vi "Drive_Auto_Module.vi"(5 "Y":dbl, 6 "Delay (s)":dbl, 7 "X":dbl, 11 "DevRef&Err":T7) -> (3 "DevRef&Err":T7)   [LabVIEW 2017]
uses:
  <vilib>/Rock Robotics/WPI/RobotDrive/WPI_RobotDriveDevRef.ctl
  <vilib>/Rock Robotics/WPI/MotorControl/WPI_MotorControlDeviceRef.ctl
  <vilib>/Rock Robotics/WPI/MotorControl/WPI_MotorControlType.ctl
  <vilib>/Rock Robotics/SystemInterfaces/DIO/FPGA_DIOPWMChannel.ctl
  <vilib>/Rock Robotics/WPI/PWM/WPI_PWMDeadband.ctl
  <vilib>/Rock Robotics/SystemInterfaces/DIO/FPGA_DIOChannel.ctl
  <vilib>/Rock Robotics/WPI/RobotDrive/WPI_RobotDriveMecanumDrive_Cartesian.vi
  <vilib>/Rock Robotics/Network Tables/NT Write Numeric Array.vi
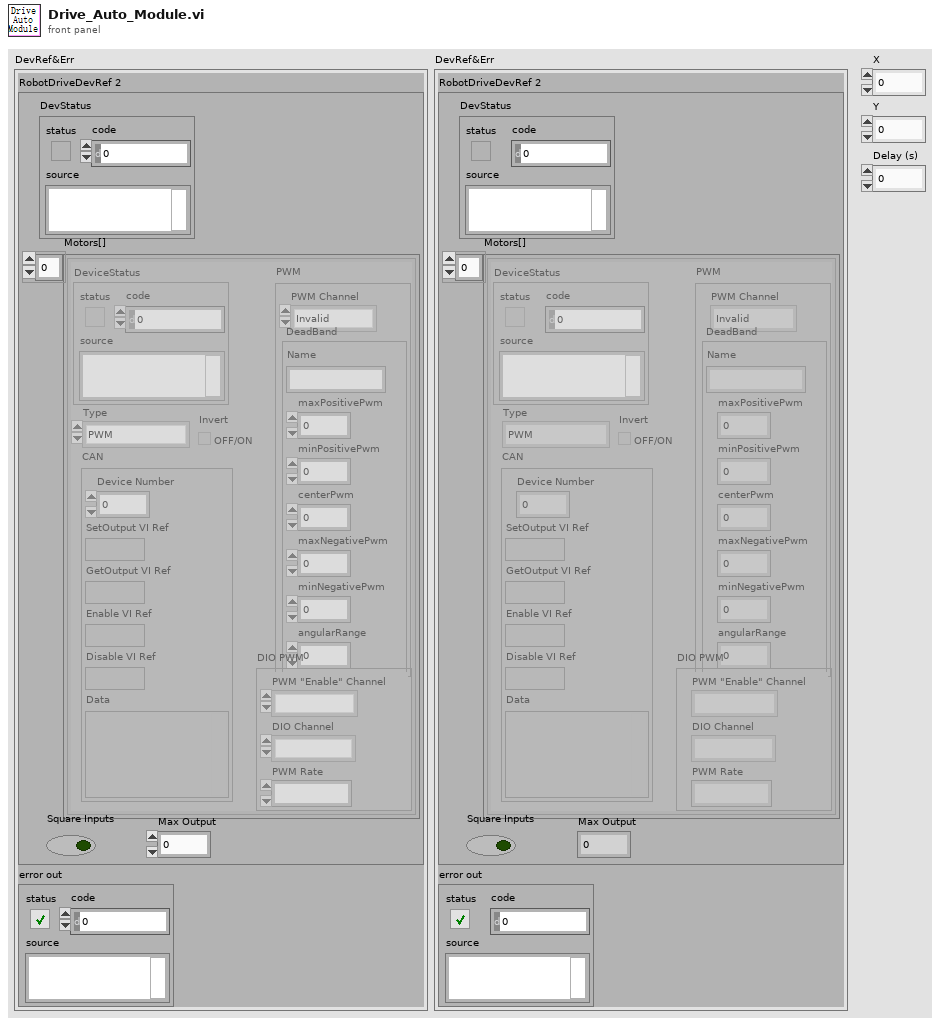
[diagram p1: front panel]
types:
  T1 = typedef "WPI_RobotDriveDevRef.ctl" = cluster{"DevStatus":errorcluster, "Motors[]":T2[], "Square Inputs":bool, "Max Output":dbl}
  T2 = typedef "WPI_MotorControlDeviceRef.ctl" = cluster{"DeviceStatus":errorcluster, "Type":T3, "PWM":cluster{"PWM Channel":T4, "DeadBand":T5}, "CAN":cluster{"Device Number":u8, "SetOutput VI Ref":variant, "GetOutput VI Ref":variant, "Enable VI Ref":variant, "Disable VI Ref":variant, "Data":variant}, "Invert":bool, "DIO PWM":cluster{"PWM \"Enable\" Channel":T4, "DIOChannel":T6, "PWM Rate":dbl}}
  T3 = typedef "WPI_MotorControlType.ctl" = enum16{"PWM", "CAN", "DIO PWM"}
  T4 = typedef "FPGA_DIOPWMChannel.ctl" = enum8{"PWM 0", "PWM 1", "PWM 2", "PWM 3", "PWM 4", "PWM 5", "PWM 6", "PWM 7", "PWM 8", "PWM 9", "PWM MXP 0", "PWM MXP 1", "PWM MXP 2", "PWM MXP 3", "PWM MXP 4", "PWM MXP 5", "PWM MXP 6", "PWM MXP 7", "PWM MXP 8", "PWM MXP 9", "Invalid"}
  T5 = typedef "WPI_PWMDeadband.ctl" = cluster{"Name":string, "maxPositivePwm":i32, "minPositivePwm":i32, "centerPwm":i32, "maxNegativePwm":i32, "minNegativePwm":i32, "angularRange":u16}
  T6 = typedef "FPGA_DIOChannel.ctl" = enum8{"DIO 0", "DIO 1", "DIO 2", "DIO 3", "DIO 4", "DIO 5", "DIO 6", "DIO 7", "DIO 8", "DIO 9", "DIO MXP 0", "DIO MXP 1", "DIO MXP 2", "DIO MXP 3", "DIO MXP 4", "DIO MXP 5", "DIO MXP 6", "DIO MXP 7", "DIO MXP 8", "DIO MXP 9", "DIO MXP 10", "DIO MXP 11", "DIO MXP 12", "DIO MXP 13", "DIO MXP 14", "DIO MXP 15", "SPI Port CS1", "SPI Port CS2", "SPI Port CS3", "SPI Port MISO", "SPI Port MOSI", "Invalid"}
  T7 = cluster{"RobotDriveDevRef 2":T1, "error out":errorcluster}
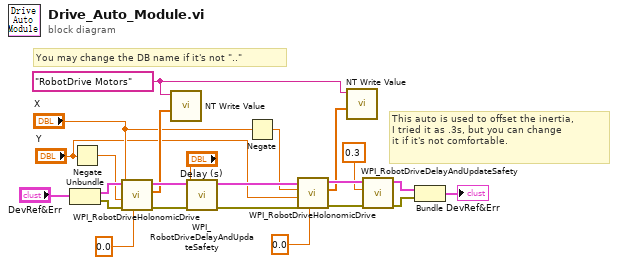
[diagram p0: block diagram]
diagram:
  w9 = "RobotDrive Motors" ("Name")
  # "You may change the DB name if it's not \"..\""
  # "This auto is used to offset the inertia,\nI tried it as .3s, but you can change\nit if it's not comfortable."
  n1 = Unbundle("DevRef&Err") -> ("RobotDriveDevRef 2"=w18:T1, "error out"=w19:errorcluster)
  n2 = Negate(x="Y") -> (-x=w2:dbl)
  n3 = call-poly <vilib>:"WPI_RobotDriveHolonomicDrive.vi"("Rotation"=0.0, "error in (no error)"=w19, "Y"=w2, "X"="X", "RobotDriveDevRef"=w18) -> ("error out"=w23:errorcluster, "Motor Values"=w16:dbl[], "RobotDriveDevRef"=w21:T1)  [unwired: 4 in]
  n4 = call-poly <vilib>:"NT Write Value.vi"("Numeric Array"=w16, "Name"=w9) -> ()  [unwired: 9 in, 1 out]
  n5 = call <vilib>:"WPI_RobotDriveDelayAndUpdateSafety.vi"("error in (no error)"=w23, "Delay (s)"="Delay (s)", "RobotDriveDevRef"=w21) -> ("error out"=w7:errorcluster, "RobotDriveDevRef 2"=w8:T1)  [unwired: 7 in]
  n6 = Negate(x="X") -> (-x=w3:dbl)
  n7 = call-poly <vilib>:"WPI_RobotDriveHolonomicDrive.vi"("Rotation"=0.0, "error in (no error)"=w7, "Y"="Y", "X"=w3, "RobotDriveDevRef"=w8) -> ("error out"=w14:errorcluster, "Motor Values"=w12:dbl[], "RobotDriveDevRef"=w13:T1)  [unwired: 4 in]
  n8 = call-poly <vilib>:"NT Write Value.vi"("Numeric Array"=w12, "Name"=w9) -> ()  [unwired: 9 in, 1 out]
  n9 = call <vilib>:"WPI_RobotDriveDelayAndUpdateSafety.vi"("error in (no error)"=w14, "Delay (s)"=0.3, "RobotDriveDevRef"=w13) -> ("error out"=w5:errorcluster, "RobotDriveDevRef 2"=w6:T1)  [unwired: 7 in]
  n10 = Bundle("RobotDriveDevRef 2"=w6, "error out"=w5) -> (→"DevRef&Err":T7)  [unwired: 1 in]
